vi "DataToFile.vi"(8 "error in (no error)":errorcluster, 10 "Sensor Index/\nSegment No.":u32, 11 "File Refnum in":refnum<file>) -> (0 "error out":errorcluster, 3 "File Refnum out":refnum<file>)   [LabVIEW 2013]
uses:
  globals/QC_RunInformation.vi
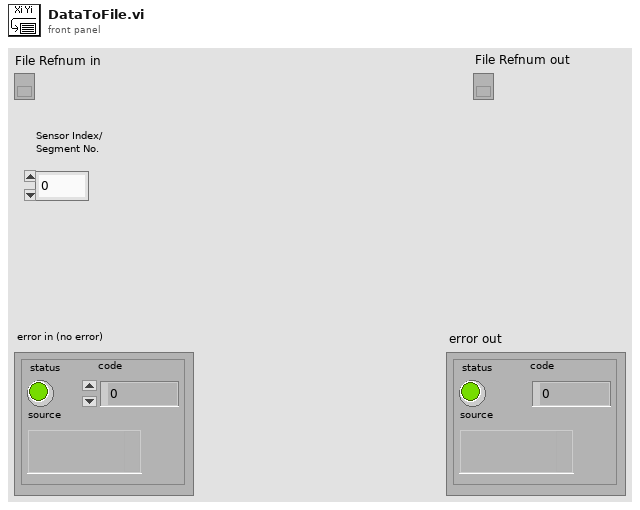
[diagram p1: front panel]
types:
  T1 = enum16{"Reset", "Read Array", "Read Element", "Write Element", "Write Array", "Add Element", "Add Array"}
  T2 = cluster{"Sensor Serial No.:":string, "Wafer:":string, "Batch:":string, "Manufacturer:":string, "Device Category:":string, "Database Serial No.:":string, "Date Initiated:":string, "Time Initiated:":string, "Test":string, "Probeplan used:":string, "End of Run comment:":string, "User:":string, "Vbias SMU":string, "LCR":string, "Test SMU":string, "Test DMM":string}
  T3 = cluster{"Current Data":u32, "Data OUT":dbl, "Data OUT":dbl, "Data OUT":dbl}[]
  T4 = cluster{"Data OUT":dbl, "Data OUT":dbl, "Data OUT":dbl, dbl}[]
  T5 = cluster{"Data OUT":dbl, "Data OUT":dbl, "Data OUT":dbl}[]
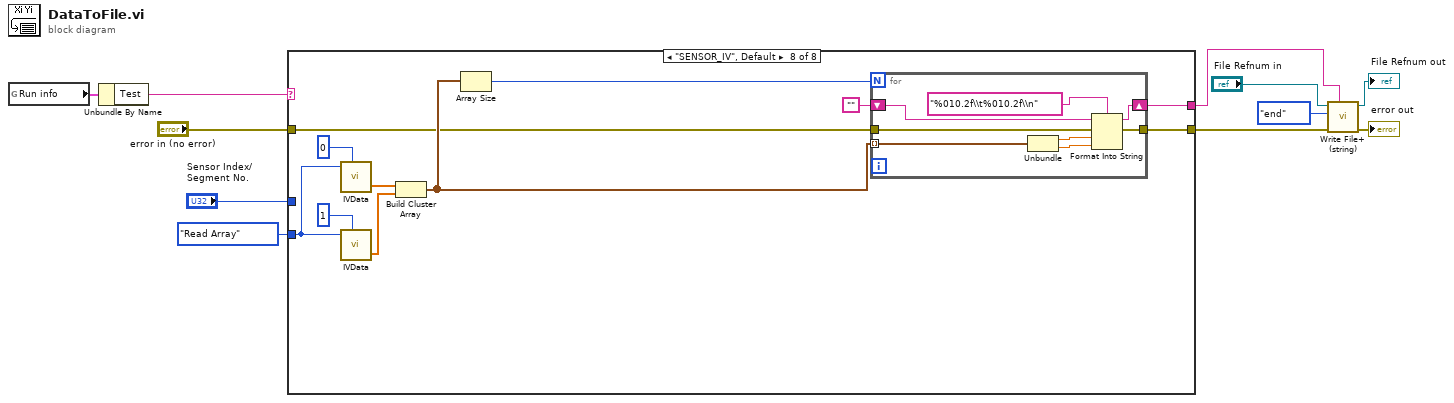
[diagram p0: block diagram]
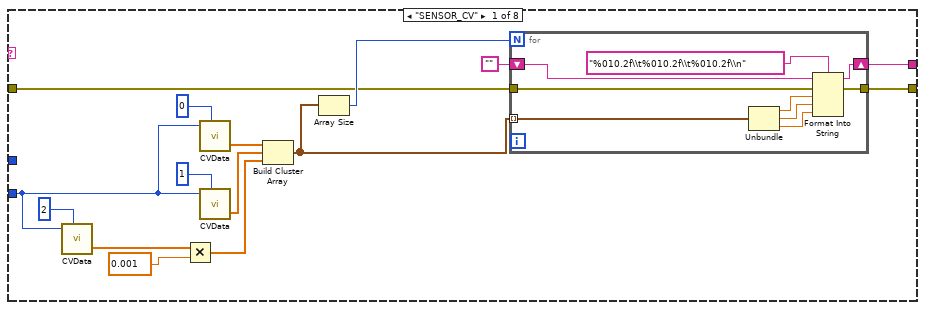
[diagram p2: hidden frame]
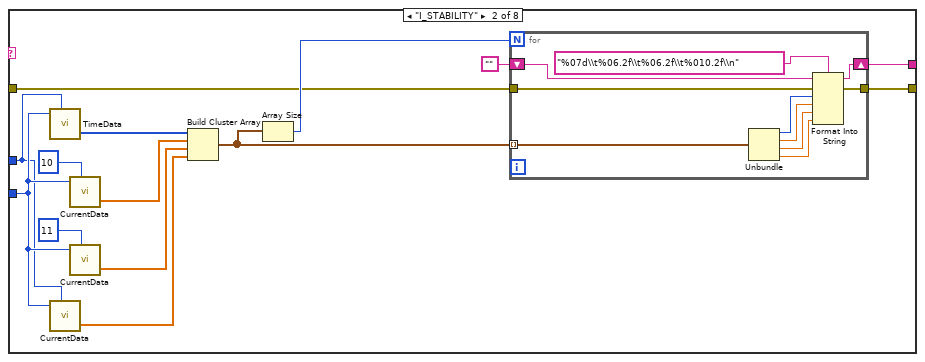
[diagram p3: hidden frame]
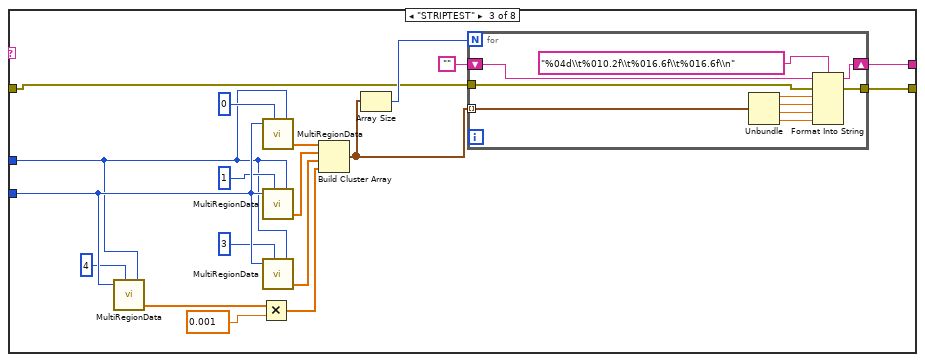
[diagram p4: hidden frame]
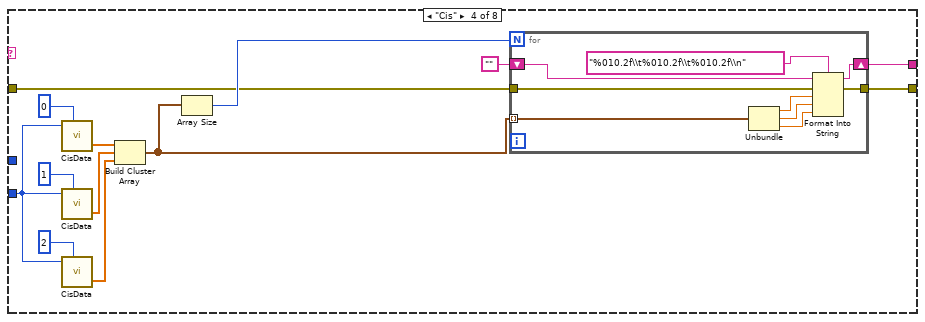
[diagram p5: hidden frame]
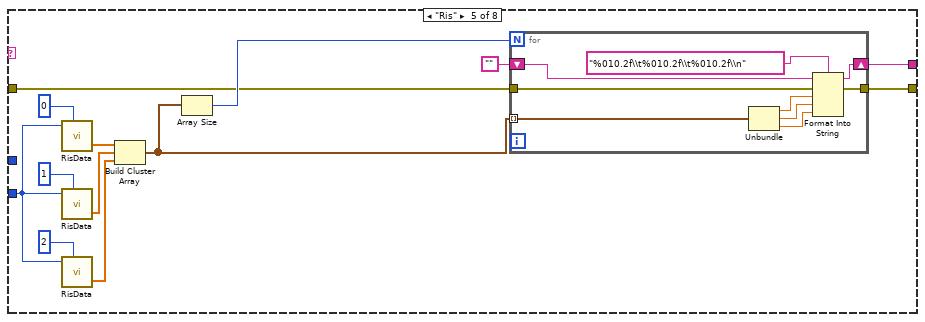
[diagram p6: hidden frame]
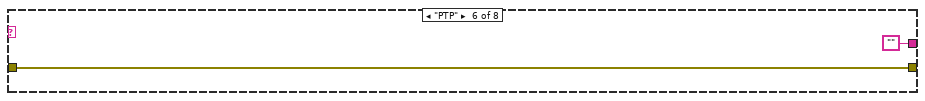
[diagram p7: hidden frame]
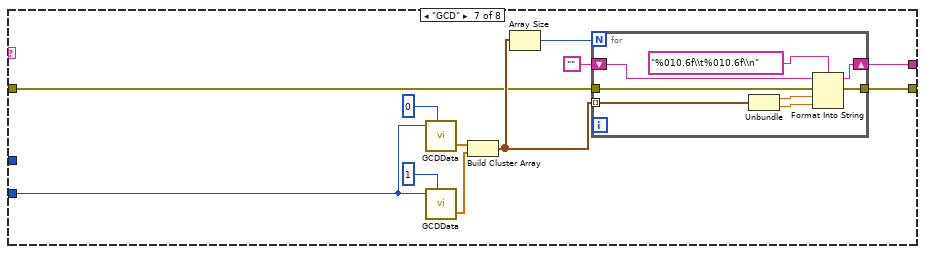
[diagram p8: hidden frame]
diagram:
  n1 = global read "QC_RunInformation.vi" "Run info"() -> (w11:T2)
  n2 = Unbundle By Name(w11) -> ("Test"=w10:string)
  n3 = case shown="\"SENSOR_IV\", Default" w10 {
    tunnel: T1."Read Array" ("Action") -> [w22 w47 w77 w91 w119 _ w140 w163]
    tunnel: [w16 w39 w62 w90 w111 "" w134 w156] -> w5
    tunnel: "error in (no error)" -> [w24 w41 w64 w98 w113 w132 w137 w155]
    tunnel: [w17 w40 w63 w89 w112 w132 w136 w154] -> w3
    tunnel: "Sensor Index/\nSegment No." -> [_ w37 w61 _ _ _ _ _]
    frame "SENSOR_CV" {
      n4 = call "CVData.vi"("Action"=w22, "Array No."=u32 2 ("Action")) -> ("Array OUT"=w14:dbl[])  [unwired: 3 in, 1 out]
      n5 = Multiply(x=w14, y=0.001) -> (x*y=w13:dbl[])
      n6 = call "CVData.vi"("Action"=w22, "Array No."=u32 0 ("Action")) -> ("Array OUT"=w18:dbl[])  [unwired: 3 in, 1 out]
      n7 = call "CVData.vi"("Action"=w22, "Array No."=u32 1 ("Action")) -> ("Array OUT"=w19:dbl[])  [unwired: 3 in, 1 out]
      n8 = Build Cluster Array(w18, w19, w13) -> (w26:cluster{"Data OUT":dbl, "Data OUT":dbl, dbl}[])
      n9 = Array Size(array=w26) -> (size(s)=w25:i32)
      n10 = for {
        N: w25 -> [_]
        tunnel: w26 -> [w35] mode=indexing
        tunnel: w24 -> [w30]
        tunnel: [w29] -> w17
        shift-right: [w31] -> w16
        shift-left: "" -> [w28]
        n11 = Unbundle(w35) -> ("Data OUT"=w34:dbl, "Data OUT"=w33:dbl, w27:dbl)
        n12 = Format Into String(format string="%010.2f\\t%010.2f\\t%010.2f\\n", initial string=w28, error in=w30, w34, w33, w27) -> (resulting string=w31:string, error out=w29:errorcluster)
      }
    }
    frame "I_STABILITY" {
      n13 = call "TimeData.vi"("Action"=w47, "Array No."=w37) -> ("Array OUT"=w44:u32[])  [unwired: 3 in, 1 out]
      n14 = call "CurrentData.vi"("Action"=w47, "Array No."=w37) -> ("Array OUT"=w38:dbl[])  [unwired: 3 in, 1 out]
      n15 = call "CurrentData.vi"("Action"=w47, "Array No."=u32 10 ("Action")) -> ("Array OUT"=w43:dbl[])  [unwired: 3 in, 1 out]
      n16 = call "CurrentData.vi"("Action"=w47, "Array No."=u32 11 ("Action")) -> ("Array OUT"=w42:dbl[])  [unwired: 3 in, 1 out]
      n17 = Build Cluster Array(w44, w43, w42, w38) -> (w49:T3)
      n18 = Array Size(array=w49) -> (size(s)=w48:i32)
      n19 = for {
        N: w48 -> [_]
        tunnel: w49 -> [w59] mode=indexing
        tunnel: w41 -> [w54]
        tunnel: [w53] -> w40
        shift-right: [w55] -> w39
        shift-left: "" -> [w52]
        n20 = Unbundle(w59) -> ("Current Data"=w58:u32, "Data OUT"=w57:dbl, "Data OUT"=w51:dbl, "Data OUT"=w50:dbl)
        n21 = Format Into String(format string="%07d\\t%06.2f\\t%06.2f\\t%010.2f\\n", initial string=w52, error in=w54, w58, w57, w51, w50) -> (resulting string=w55:string, error out=w53:errorcluster)
      }
    }
    frame "STRIPTEST" {
      n22 = call "MultiRegionData.vi"("Action"=w77, "Array No."=u32 4 ("Action"), "Region index"=w61) -> ("Array OUT"=w71:dbl[])  [unwired: 3 in, 1 out]
      n23 = Multiply(x=w71, y=0.001) -> (x*y=w65:dbl[])
      n24 = call "MultiRegionData.vi"("Action"=w77, "Array No."=u32 0 ("Action"), "Region index"=w61) -> ("Array OUT"=w68:dbl[])  [unwired: 3 in, 1 out]
      n25 = call "MultiRegionData.vi"("Action"=w77, "Array No."=u32 1 ("Action"), "Region index"=w61) -> ("Array OUT"=w67:dbl[])  [unwired: 3 in, 1 out]
      n26 = call "MultiRegionData.vi"("Action"=w77, "Array No."=u32 3 ("Action"), "Region index"=w61) -> ("Array OUT"=w66:dbl[])  [unwired: 3 in, 1 out]
      n27 = Build Cluster Array(w68, w67, w66, w65) -> (w70:T4)
      n28 = Array Size(array=w70) -> (size(s)=w69:i32)
      n29 = for {
        N: w69 -> [_]
        tunnel: w70 -> [w87] mode=indexing
        tunnel: w64 -> [w82]
        tunnel: [w81] -> w63
        shift-right: [w83] -> w62
        shift-left: "" -> [w80]
        n30 = Unbundle(w87) -> ("Data OUT"=w86:dbl, "Data OUT"=w85:dbl, "Data OUT"=w79:dbl, w78:dbl)
        n31 = Format Into String(format string="%04d\\t%010.2f\\t%016.6f\\t%016.6f\\n", initial string=w80, error in=w82, w86, w85, w79, w78) -> (resulting string=w83:string, error out=w81:errorcluster)
      }
    }
    frame "Cis" {
      n32 = call "CisData.vi"("Action"=w91, "Array No."=u32 0 ("Action")) -> ("Array OUT"=w97:dbl[])  [unwired: 3 in, 1 out]
      n33 = call "CisData.vi"("Action"=w91, "Array No."=u32 1 ("Action")) -> ("Array OUT"=w96:dbl[])  [unwired: 3 in, 1 out]
      n34 = call "CisData.vi"("Action"=w91, "Array No."=u32 2 ("Action")) -> ("Array OUT"=w95:dbl[])  [unwired: 3 in, 1 out]
      n35 = Build Cluster Array(w97, w96, w95) -> (w100:T5)
      n36 = Array Size(array=w100) -> (size(s)=w99:i32)
      n37 = for {
        N: w99 -> [_]
        tunnel: w100 -> [w109] mode=indexing
        tunnel: w98 -> [w104]
        tunnel: [w103] -> w89
        shift-right: [w105] -> w90
        shift-left: "" -> [w102]
        n38 = Unbundle(w109) -> ("Data OUT"=w108:dbl, "Data OUT"=w107:dbl, "Data OUT"=w101:dbl)
        n39 = Format Into String(format string="%010.2f\\t%010.2f\\t%010.2f\\n", initial string=w102, error in=w104, w108, w107, w101) -> (resulting string=w105:string, error out=w103:errorcluster)
      }
    }
    frame "Ris" {
      n40 = call "RisData.vi"("Action"=w119, "Array No."=u32 0 ("Action")) -> ("Array OUT"=w116:dbl[])  [unwired: 3 in, 1 out]
      n41 = call "RisData.vi"("Action"=w119, "Array No."=u32 1 ("Action")) -> ("Array OUT"=w115:dbl[])  [unwired: 3 in, 1 out]
      n42 = call "RisData.vi"("Action"=w119, "Array No."=u32 2 ("Action")) -> ("Array OUT"=w114:dbl[])  [unwired: 3 in, 1 out]
      n43 = Build Cluster Array(w116, w115, w114) -> (w118:T5)
      n44 = Array Size(array=w118) -> (size(s)=w117:i32)
      n45 = for {
        N: w117 -> [_]
        tunnel: w118 -> [w131] mode=indexing
        tunnel: w113 -> [w126]
        tunnel: [w125] -> w112
        shift-right: [w127] -> w111
        shift-left: "" -> [w124]
        n46 = Unbundle(w131) -> ("Data OUT"=w130:dbl, "Data OUT"=w129:dbl, "Data OUT"=w123:dbl)
        n47 = Format Into String(format string="%010.2f\\t%010.2f\\t%010.2f\\n", initial string=w124, error in=w126, w130, w129, w123) -> (resulting string=w127:string, error out=w125:errorcluster)
      }
    }
    frame "PTP" {
    }
    frame "GCD" {
      n48 = call "GCDData.vi"("Action"=w140, "Array No."=u32 0 ("Action")) -> ("Array OUT"=w138:dbl[])  [unwired: 3 in, 1 out]
      n49 = call "GCDData.vi"("Action"=w140, "Array No."=u32 1 ("Action")) -> ("Array OUT"=w139:dbl[])  [unwired: 3 in, 1 out]
      n50 = Build Cluster Array(w138, w139) -> (w144:cluster{"Data OUT":dbl, "Data OUT":dbl}[])
      n51 = Array Size(array=w144) -> (size(s)=w143:i32)
      n52 = for {
        N: w143 -> [_]
        tunnel: w144 -> [w152] mode=indexing
        tunnel: w137 -> [w147]
        tunnel: [w146] -> w136
        shift-right: [w148] -> w134
        shift-left: "" -> [w145]
        n53 = Unbundle(w152) -> ("Data OUT"=w151:dbl, "Data OUT"=w150:dbl)
        n54 = Format Into String(format string="%010.6f\\t%010.6f\\n", initial string=w145, error in=w147, w151, w150) -> (resulting string=w148:string, error out=w146:errorcluster)
      }
    }
    frame "SENSOR_IV", Default {
      n55 = call "IVData.vi"("Action"=w163, "Array No."=u32 0 ("Action")) -> ("Array OUT"=w160:dbl[])  [unwired: 3 in, 1 out]
      n56 = call "IVData.vi"("Action"=w163, "Array No."=u32 1 ("Action")) -> ("Array OUT"=w159:dbl[])  [unwired: 3 in, 1 out]
      n57 = Build Cluster Array(w160, w159) -> (w158:cluster{"Data OUT":dbl, "Data OUT":dbl}[])
      n58 = Array Size(array=w158) -> (size(s)=w157:i32)
      n59 = for {
        N: w157 -> [_]
        tunnel: w158 -> [w171] mode=indexing
        tunnel: w155 -> [w166]
        tunnel: [w165] -> w154
        shift-right: [w167] -> w156
        shift-left: "" -> [w164]
        n60 = Unbundle(w171) -> ("Data OUT"=w170:dbl, "Data OUT"=w169:dbl)
        n61 = Format Into String(format string="%010.2f\\t%010.2f\\n", initial string=w164, error in=w166, w170, w169) -> (resulting string=w167:string, error out=w165:errorcluster)
      }
    }
  }
  n62 = call <vilib>:"Write File+ (string).vi"("string"=w5, "error in (no error)"=w3, "pos mode (rel. to end:1)"=enum16{"start", "end", "current"}."end", "refnum"="File Refnum in") -> ("error out"=→"error out":errorcluster, "dup refnum"=→"File Refnum out":refnum<file>)  [unwired: 3 in, 1 out]
